vi "acq.constructImage.EL.vi"(7 "DVR":T1, 8 "error in":errorcluster, 10 "queue1 in":refnum<queue>) -> (0 "error out":errorcluster, 2 "EL":u16[][](array[numeric]))   [LabVIEW 2020]
uses:
  _controls/data.ref.ctl
  _controls/state.ctl
  _controls/data.vars.ctl
  _controls/data.ctl
  _controls/flip.ctl
  <vilib>/vision/Image Controls.llb/IMAQ Image.ctl
  camera/camera.lvclass
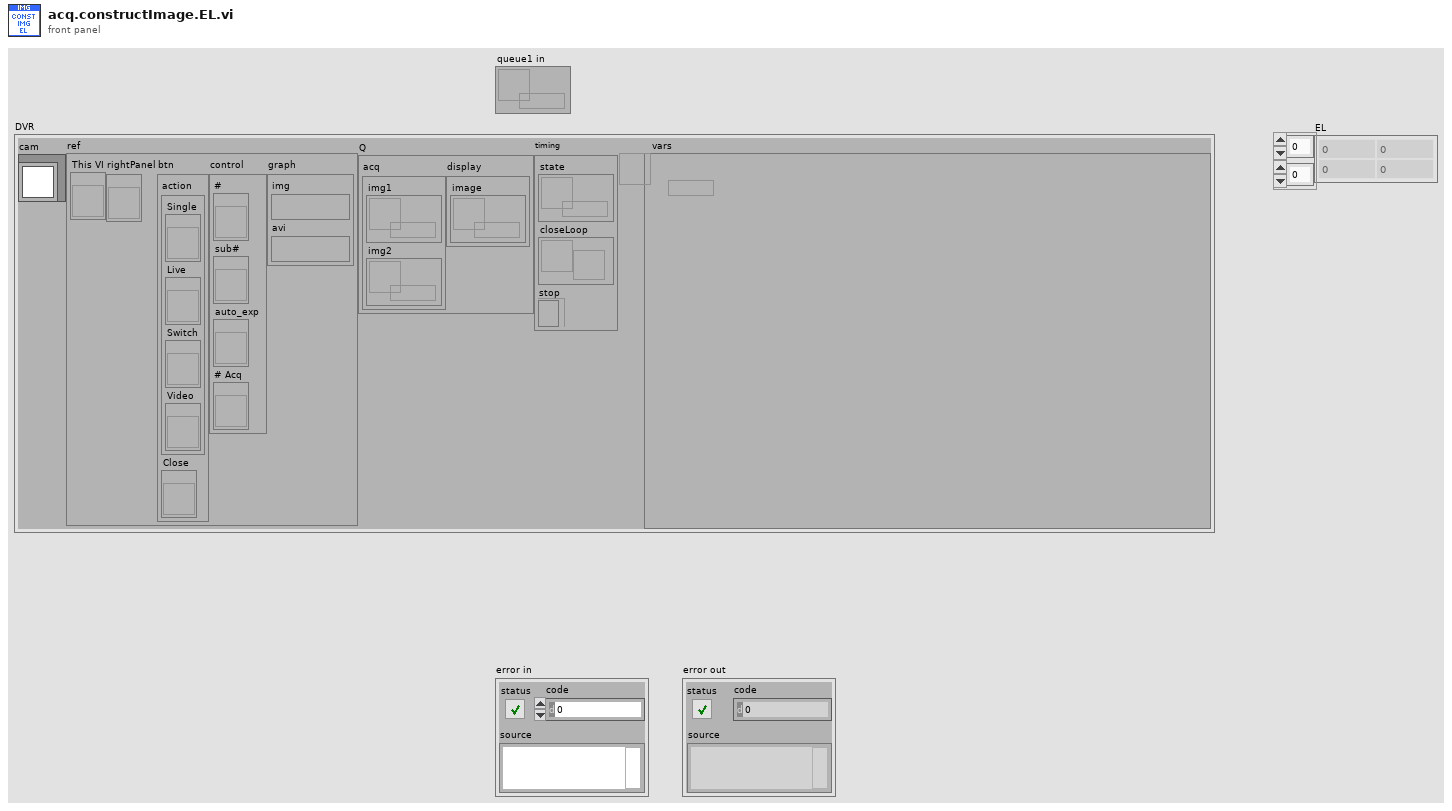
[diagram p1: front panel]
types:
  T1 = typedef "data.ctl" = cluster{"cam":refnum<class "camera.lvclass">, "ref":T2, "Q":cluster{"acq":cluster{"img1":refnum<queue>, "img2":refnum<queue>}, "display":cluster{"image":refnum<queue>}}, "timing":cluster{"state":refnum<queue>, "closeLoop":refnum<notifier>, "stop":refnum<k4>}, "vars":refnum<data-value>}
  T2 = typedef "data.ref.ctl" = cluster{"This VI":refnum<vi>, "rightPanel":refnum<vi>, "btn":cluster{"action":cluster{"Single":refnum<vi>, "Live":refnum<vi>, "Switch":refnum<vi>, "Video":refnum<vi>}, "Close":refnum<vi>}, "control":cluster{"#":refnum<vi>, "sub#":refnum<vi>, "auto_exp":refnum<vi>, "# Acq":refnum<vi>}, "graph":cluster{"img":T3, "avi":T3}}
  T3 = typedef "IMAQ Image.ctl" = refnum<image>
  T4 = typedef "data.vars.ctl" = cluster{"save":cluster{"base_folder":cluster{"Folder":path, "tif":bool, "jpg":bool}, "module":string, "#":u32, "sub#":u8, "save.op":enum16{"Full", "Light"}, "same?":bool, "Shift":enum16{"Single", "Leapfrog"}, "jpg?":bool, "flip":T5}, "acq":cluster{"# Acq":u16, "rotate":bool, "FPS":dbl}, "calib.manual":cluster{"BG":cluster{"Image":u16[][], "enabled?":bool}, "FF":cluster{"Image":u16[][], "enabled?":bool}}}
  T5 = typedef "flip.ctl" = cluster{"x":bool, "y":bool}
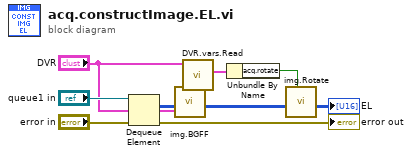
[diagram p0: block diagram]
diagram:
  n1 = Dequeue Element(queue="queue1 in", error in (no error)="error in") -> (element=w6:u16[][], error out=→"error out":errorcluster)  [unwired: 1 in, 2 out]
  n2 = call "img.BGFF.vi"("DVR"="DVR", "image in"=w6) -> ("image out"=w2:u16[][])  [unwired: 9 in]
  "EL" <- w2
  n3 = call "DVR.vars.Read.vi"("DVR.state"="DVR") -> ("vars"=w5:T4)  [unwired: 9 in, 1 out]
  n4 = Unbundle By Name(w5) -> ("acq.rotate"=w3:bool)
  n5 = call "img.Rotate.vi"("rotate"=w3, "image in"=w2) -> ()  [unwired: 9 in, 1 out]
